vi "Convert-I16-to-FXP.vi"(5 "Overflow":bool, 6 "I16 in":i16) -> (2 "data out":T1)   [LabVIEW 2015, in "DDC_7976R_v1.lvlib"]
uses:
  DDC_7976R_v1.lvlib
  <instrlib>/_niInstr/DSP/v1/Shared/Public/IQ Data.ctl
  <vilib>/rvi/FXPMathLib/FxpConvert/subVIs/nifxpmath_Convert_SimConfig.ctl
  <vilib>/fxp/LVFixedPointQuantizationPolicyTypeDef.ctl
  <vilib>/fxp/LVFixedPointOverflowPolicyTypeDef.ctl
  <vilib>/rvi/FXPMathLib/FxpConvert/simVIs/DllFxpConvertTemp_sub.vi
  <vilib>/rvi/FXPMathLib/FxpConvert/XNode/nifxpmath_Convert.xnode
  <vilib>/rvi/FXPMathLib/FxpInterpret/XNode/nifxpmath_Interpret.xnode
  <instrlib>/_niInstr/DSP/v1/Shared/niInstr DSP v1 Shared.lvlib
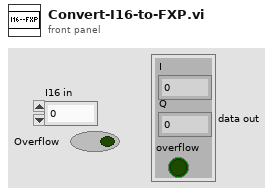
[diagram p1: front panel]
types:
  T1 = typedef "niInstr DSP v1 Shared.lvlib/IQ Data.ctl" = cluster{"I":fxp<+/-,18,1>, "Q":fxp<+/-,18,1>, "overflow":bool}
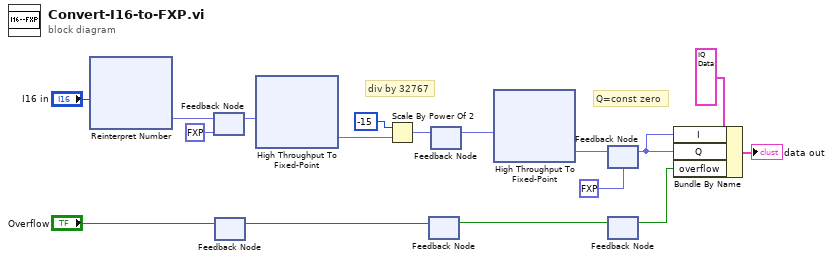
[diagram p0: block diagram]
diagram:
  # "Q=const zero"
  # "div by 32767"
  n1 = xnode "Reinterpret Number"("x"="I16 in") -> ("y"=w10:fxp<+/-,16,16>)
  n2 = feedback-in #1(w10) -> ()
  n3 = feedback #1(fxp<+/-,16,16> 0.0 ("y")) -> (w9:fxp<+/-,16,16>)
  n4 = feedback #2() -> (w13:bool)  [unwired: 1 in]
  n5 = feedback-in #2("Overflow") -> ()
  n6 = xnode "High Throughput To Fixed-Point"("x"=w9) -> ("y"=w8:fxp<+/-,36,18>)
  n7 = Scale By Power Of 2(n=i16 -15, x=w8) -> (x*2^n=w3:fxp<+/-,36,18>)
  n8 = feedback #3() -> (w5:bool)  [unwired: 1 in]
  n9 = feedback-in #3(w13) -> ()
  n10 = feedback #4() -> (w2:fxp<+/-,36,18>)  [unwired: 1 in]
  n11 = feedback-in #4(w3) -> ()
  n12 = xnode "High Throughput To Fixed-Point"("x"=w2) -> ("y"=w6:fxp<+/-,18,1>)
  n13 = feedback #5(fxp<+/-,18,1> 0.0 ("y")) -> (w1:fxp<+/-,18,1>)
  n14 = feedback-in #5(w6) -> ()
  n15 = feedback #6() -> (w4:bool)  [unwired: 1 in]
  n16 = feedback-in #6(w5) -> ()
  n17 = Bundle By Name(cluster=T1 {"I"=0.0, "Q"=0.0, "overflow"=FALSE} ("data"), "I"=w1, "Q"=w1, "overflow"=w4) -> (→"data out":T1)
